vi "lvUpdateProjectFiles.vi"() -> ()   [LabVIEW 2015, in "veristand-steps-build-tools.lvlib"]
uses:
  veristand-steps-build-tools.lvlib
panel:
  out "error out":errorcluster
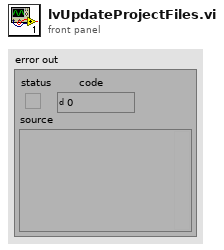
[diagram p1: front panel]
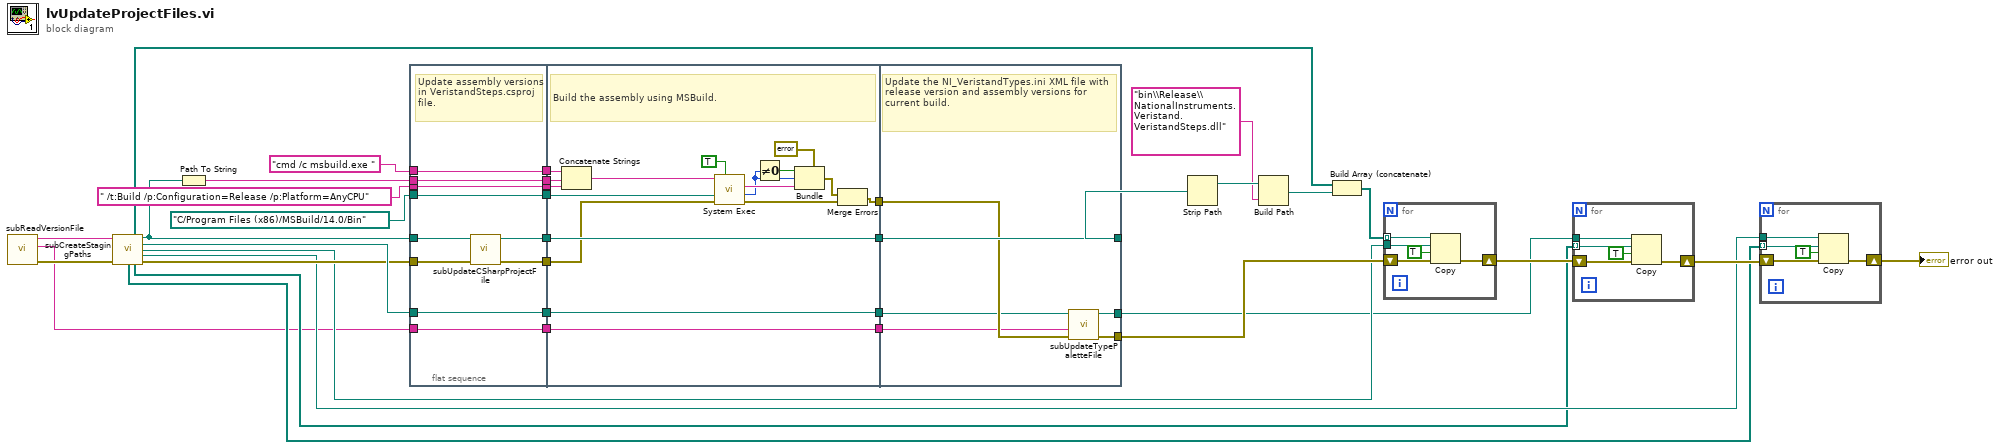
[diagram p0: block diagram]
diagram:
  n1 = call "subReadVersionFile.vi"() -> ("error out"=w3:errorcluster, "Step Types Version"=w1:string, "TestStand Versions"=w2:string)  [unwired: 9 in]
  n2 = call "subCreateStagingPaths.vi"("TestStand Version String"=w2, "error in"=w3) -> ("GACUtilityPaths"=w16:path[], "CSharp Assembly Project Path"=w22:path, "TypePalette File Path"=w19:path, "Program Files Destination Path"=w10:path, "Icon File Path"=w12:path, "Icon Paths"=w5:path[], "TypePalettes Paths"=w4:path[], "Error out"=w13:errorcluster)  [unwired: 6 in]
  n3 = Path To String(path=w22) -> (string=w21:string)
  n4 = flat-sequence {
    tunnel: " /t:Build /p:Configuration=Release /p:Platform=AnyCPU" ("string") -> [w46]
    tunnel: "cmd /c msbuild.exe " -> [w47]
    tunnel: [w47] -> w34
    tunnel: [w46] -> w33
    tunnel: w22 -> [w45]
    tunnel: [w44] -> w32
    tunnel: [w43] -> w31
    tunnel: w21 -> [w42]
    tunnel: [w42] -> w20
    tunnel: w19 -> [w41]
    tunnel: [w41] -> w17
    tunnel: w1 -> [w40]
    tunnel: [w40] -> w15
    tunnel: w13 -> [w39]
    tunnel: path "C:/Program Files (x86)/MSBuild/14.0/Bin" ("working directory") -> [w38]
    tunnel: [w38] -> w6
    tunnel: [w64] -> w29
    tunnel: w31 -> [w64]
    tunnel: w32 -> [w59]
    tunnel: w33 -> [w61]
    tunnel: w34 -> [w62]
    tunnel: [w49] -> w28
    tunnel: w20 -> [w58]
    tunnel: [w57] -> w18
    tunnel: w17 -> [w57]
    tunnel: w15 -> [w56]
    tunnel: [w56] -> w14
    tunnel: w6 -> [w48]
    tunnel: [w70] -> w11
    tunnel: w29 -> [w70]
    tunnel: [w69] -> w27
    tunnel: w28 -> [w68]
    tunnel: w18 -> [w66]
    tunnel: w14 -> [w67]
    tunnel: [w65] -> w9
    frame #0 {
      # "Update assembly versions in VeristandSteps.csproj file."
      n5 = call "subUpdateCSharpProjectFile.vi"("error in (no error)"=w39, ".csproj path"=w45) -> ("error out"=w44:errorcluster, ".csproj path out"=w43:path)  [unwired: 8 in]
    }
    frame #1 {
      # "Build the assembly using MSBuild."
      n6 = Concatenate Strings(w62, w58, w61) -> (w60:string)
      n7 = call <vilib>:"System Exec.vi"("wait until completion? (T)"=TRUE, "error in (no error)"=w59, "working directory"=w48, "command line"=w60) -> ("error out"=w50:errorcluster, "return code"=w53:i32, "standard error"=w54:string)  [unwired: 4 in, 1 out]
      n8 = Not Equal To 0?(x=w53) -> (x != 0?=w52:bool)
      n9 = Bundle(cluster=errorcluster {"status"=FALSE, "code"=0, "source"=""} ("error constant"), "status"=w52, "code"=w53, "source"=w54) -> (w51:errorcluster)
      n10 = Merge Errors(w51, w50) -> (w49:errorcluster)
    }
    frame #2 {
      # "Update the NI_VeristandTypes.ini XML file with release version and assembly versions for current build."
      n11 = call "subUpdateTypePaletteFile.vi"("error in (no error)"=w68, "Step Types Version"=w67, "TypePalette .ini file location"=w66) -> ("error out"=w69:errorcluster, "Type Palettes File Path out"=w65:path)  [unwired: 7 in]
    }
  }
  n12 = Strip Path(path=w11) -> (stripped path=w36:path)  [unwired: 1 out]
  n13 = Build Path(base path=w36, name or relative path="bin\\Release\\NationalInstruments.Veristand.VeristandSteps.dll") -> (appended path=w26:path)
  n14 = Build Array (concatenate)(w16, w26) -> (w25:path[])
  n15 = for {
    shift-right: [w75] -> w24
    shift-left: w27 -> [w74]
    tunnel: w25 -> [w73] mode=indexing
    tunnel: w10 -> [w72]
    n16 = Copy(8:w74, 9:TRUE ("overwrite (F)"), 10:w72, 11:w73) -> (0:w75:errorcluster)  [unwired: 1 in, 2 out]
  }
  n17 = for {
    shift-right: [w80] -> w23
    shift-left: w24 -> [w79]
    tunnel: w9 -> [w77]
    tunnel: w4 -> [w76] mode=indexing
    n18 = Copy(8:w79, 9:TRUE ("overwrite (F)"), 10:w76, 11:w77) -> (0:w80:errorcluster)  [unwired: 1 in, 2 out]
  }
  n19 = for {
    shift-right: [w85] -> w8
    shift-left: w23 -> [w84]
    tunnel: w12 -> [w82]
    tunnel: w5 -> [w81] mode=indexing
    n20 = Copy(8:w84, 9:TRUE ("overwrite (F)"), 10:w81, 11:w82) -> (0:w85:errorcluster)  [unwired: 1 in, 2 out]
  }
  "error out" <- w8
